vi "Async Get image from CamServer.vi"(2 "Quality":u32=750 max=1000, 3 "Image name":string="test", 4 "Image directory path":path=path "C:/test", 5 "Camera":T1="Travcam") -> (0 "Error out":errorcluster, 1 "Image file path":path)   [LabVIEW 2015]
doc: "Asynchronously gets a snapshot image from the selected camera on the camera server and saves it to the specified path with specified name."
uses:
  Camera enum/Camera enum.ctl
  Globals/CamServer global.vi
panel:
  # "PN 21/08/15"
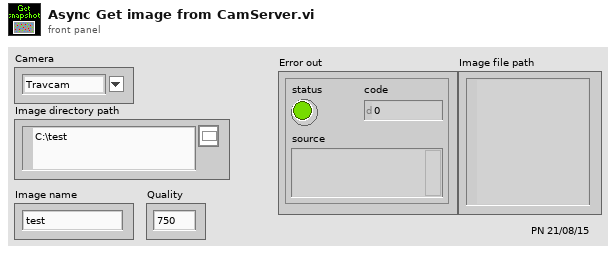
[diagram p1: front panel]
types:
  T1 = typedef "Camera enum.ctl" = string
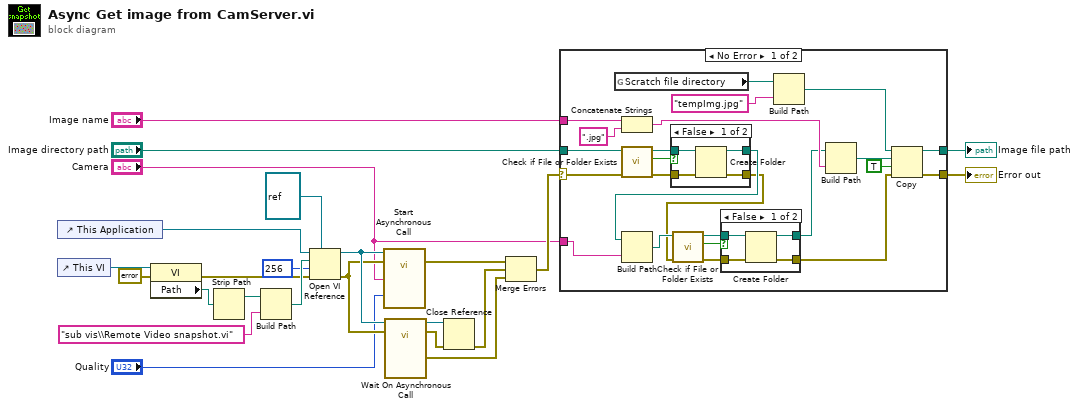
[diagram p0: block diagram]
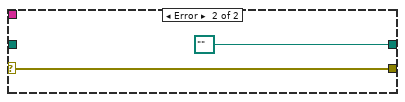
[diagram p4: hidden frame]
diagram:
  n1 = control-ref of="This Application"() -> (w19:refnum<vi>)
  n2 = control-ref of="This VI"() -> (w24:refnum<vi>)
  n3 = property class="VI"(reference=w24, error in=errorcluster {"status"=FALSE, "code"=0, "source"=""} ("error in (no error)")) -> (error out=w21:errorcluster, "Path"=w17:path)  [unwired: 1 out]
  n4 = Strip Path(path=w17) -> (stripped path=w16:path)  [unwired: 1 out]
  n5 = Build Path(base path=w16, name or relative path="sub vis\\Remote Video snapshot.vi") -> (appended path=w22:path)
  n6 = Open VI Reference(type specifier VI Refnum (for type only)=refnum<vi> refnum, application reference (local)=w19, vi path=w22, options=256, error in (no error)=w21) -> (vi reference=w15:refnum<vi>, error out=w14:errorcluster)  [unwired: 1 in]
  n7 = call-by-ref "Start Asynchronous Call"(reference=w15, error in=w14, "Quality"="Quality", "Camera"="Camera") -> (error out=w12:errorcluster)  [unwired: 2 out]
  n8 = call-by-ref "Wait On Asynchronous Call"(reference=w15, error in=w14) -> (reference out=w13:refnum<vi>, error out=w11:errorcluster, "Error out"=w9:errorcluster)  [unwired: 2 in]
  n9 = Close Reference(reference=w13, error in (no error)=w11) -> (error out=w10:errorcluster)
  n10 = Merge Errors(w12, w10, w9) -> (w5:errorcluster)
  n11 = case shown="No Error" w5 {
    selector: w5 -> [w47 w62]
    tunnel: "Image directory path" -> [w48 _]
    tunnel: "Image name" -> [w42 _]
    tunnel: [w36 w62] -> w3
    tunnel: "Camera" -> [w30 _]
    tunnel: [w25 path "" ("new path")] -> w2
    frame No Error {
      n12 = global read "CamServer global.vi" "Scratch file directory"() -> (w37:path)
      n13 = Concatenate Strings(w42, ".jpg" ("string")) -> (w40:string)
      n14 = call <vilib>:"Check if File or Folder Exists.vi"("error in (no error)"=w47, "path"=w48) -> ("error out"=w44:errorcluster, "file or folder exists?"=w46:bool, "dup path"=w45:path)  [unwired: 7 in]
      n15 = case shown="False" w46 {
        tunnel: w45 -> [w58 w60]
        tunnel: w44 -> [w57 w59]
        tunnel: [w56 w60] -> w31
        tunnel: [w55 w59] -> w28
        frame False {
          n16 = Create Folder(path (use dialog)=w58, error in=w57) -> (created path=w56:path, error out=w55:errorcluster)  [unwired: 1 in, 1 out]
        }
        frame True {
        }
      }
      n17 = Build Path(base path=w31, name or relative path=w30) -> (appended path=w29:path)
      n18 = call <vilib>:"Check if File or Folder Exists.vi"("error in (no error)"=w28, "path"=w29) -> ("error out"=w32:errorcluster, "file or folder exists?"=w33:bool, "dup path"=w34:path)  [unwired: 7 in]
      n19 = case shown="False" w33 {
        tunnel: w34 -> [w52 w54]
        tunnel: w32 -> [w51 w53]
        tunnel: [w50 w54] -> w27
        tunnel: [w49 w53] -> w26
        frame False {
          n20 = Create Folder(path (use dialog)=w52, error in=w51) -> (created path=w50:path, error out=w49:errorcluster)  [unwired: 1 in, 1 out]
        }
        frame True {
        }
      }
      n21 = Build Path(base path=w37, name or relative path="tempImg.jpg") -> (appended path=w35:path)
      n22 = Build Path(base path=w27, name or relative path=w40) -> (appended path=w41:path)
      n23 = Copy(8:w26, 9:TRUE ("overwrite (F)"), 10:w41, 11:w35) -> (0:w36:errorcluster, 3:w25:path)  [unwired: 1 in, 1 out]
    }
    frame Error {
    }
  }
  "Error out" <- w3
  "Image file path" <- w2
